vi "voltage_outer.vi"(8 "queue":refnum<queue>, 11 "Qube":refnum<class "System.lvclass">) -> (3 "Qube":refnum<class "System.lvclass">)   [LabVIEW 2021, in "System.lvclass"]
uses:
  System.lvclass
  System.lvclass/System.ctl
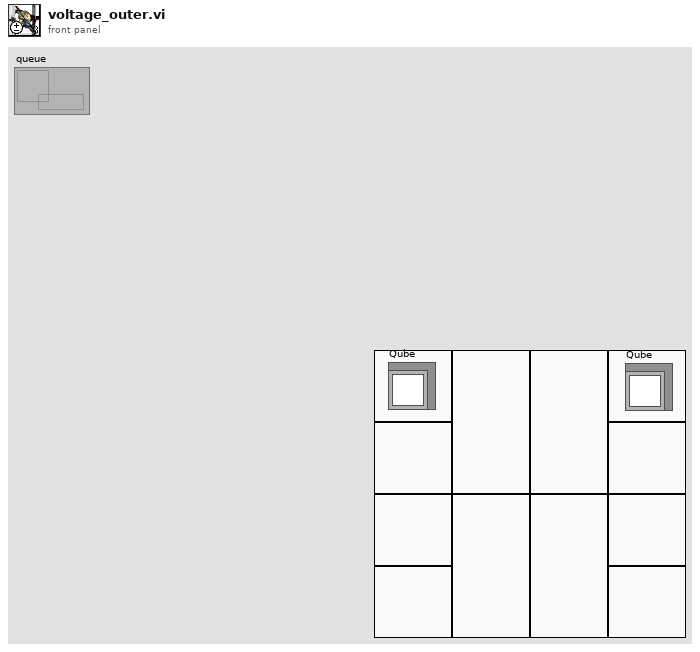
[diagram p1: front panel]
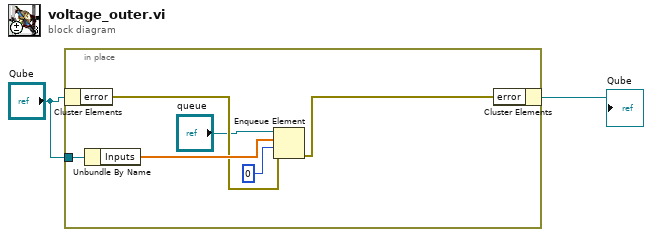
[diagram p0: block diagram]
diagram:
  n1 = in-place {
    in-place-border: "Qube" -> [w8]
    n2 = in-place-cluster #1("Qube") -> ("error"=w5:errorcluster)
    n3 = Unbundle By Name(w8) -> ("Inputs"=w7:dbl[])
    n4 = Enqueue Element(queue="queue", element=w7, timeout in ms (-1)=0, error in (no error)=w5) -> (error out=w4:errorcluster)  [unwired: 2 out]
    n5 = in-place-cluster #1("error"=w4) -> (→"Qube":refnum<class "System.lvclass">)
  }
